vi "Configure Tag Current Pulse (Linear).vi"(0 "VISA resource name":refnum<visa-resource-name>, 1 "Source Measure Unit Channel (0: Channel A)":i32(ring) items=["Channel A", "Channel B"], 2 "Bias Level (0 A)":dbl, 3 "Voltage Limit (1 V)":dbl=1.0, 4 "Voltage Buffer (smua.nvbuffer1)":string="smua.nvbuffer1", 5 "Pulse Start Level (0.01 A)":dbl=0.01, 6 "Pulse Stop Level (0.1 A)":dbl=0.1, 7 "error in (no error)":errorcluster, 8 "Pulse Train Tag (1)":i32=1, 9 "Pulse On Time (0.02 S)":dbl=0.02, 10 "Pulse Measure Cycles (10)":i32=10, 11 "Pulse Off Time (0.04 S)":dbl=0.04, 12 "Trigger Input (0)":i32, 13 "Trigger Wait Time (10 S)":dbl=10.0, 14 "Trigger Output (0)":i32, 15 "Missing Trigger (0: Nil)":i32(ring) items=["Nil", "Abort Pulse", "Not Abort Pulse"]) -> (20 "VISA resource name out":refnum<visa-resource-name>, 27 "error out":errorcluster)   [LabVIEW 2020, in "Keithley 2600 Series.lvlib"]
doc: "Configures a linear pulsed current sweep with a voltage measurement.\n\n<b>Note:</b>\nThis VI does not cause the specified source measure unit channel to output a pulse train. It simply checks to see if all the pulse dimensions can be achieved, and if they are, assigns the indicated pulse train tag to the pulse train. You need to call <b>Initiate Pulse Test </b>VI to initiate a pulse train."
uses:
  <instrlib>/Keithley 2600 Series/Keithley 2600 Series.lvlib
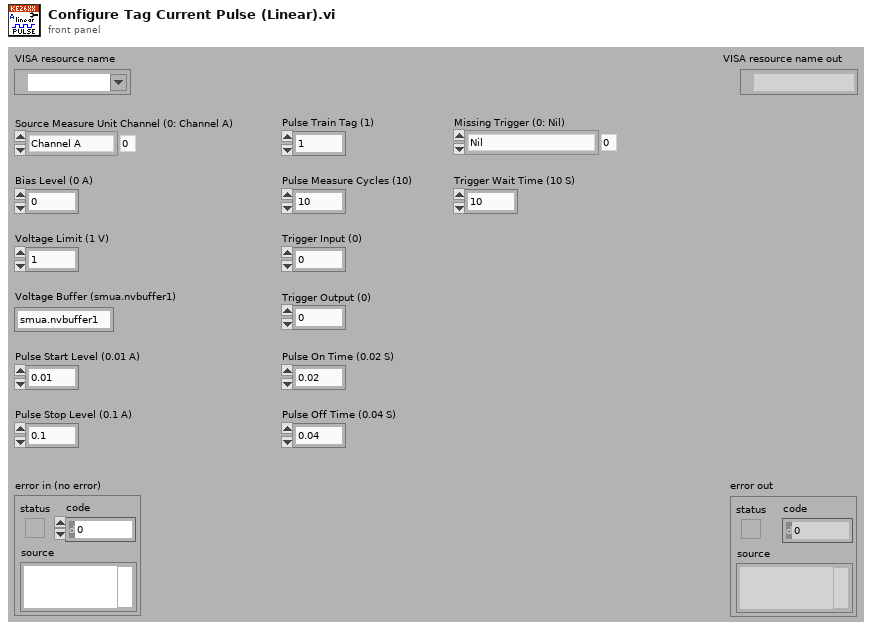
[diagram p1: front panel]
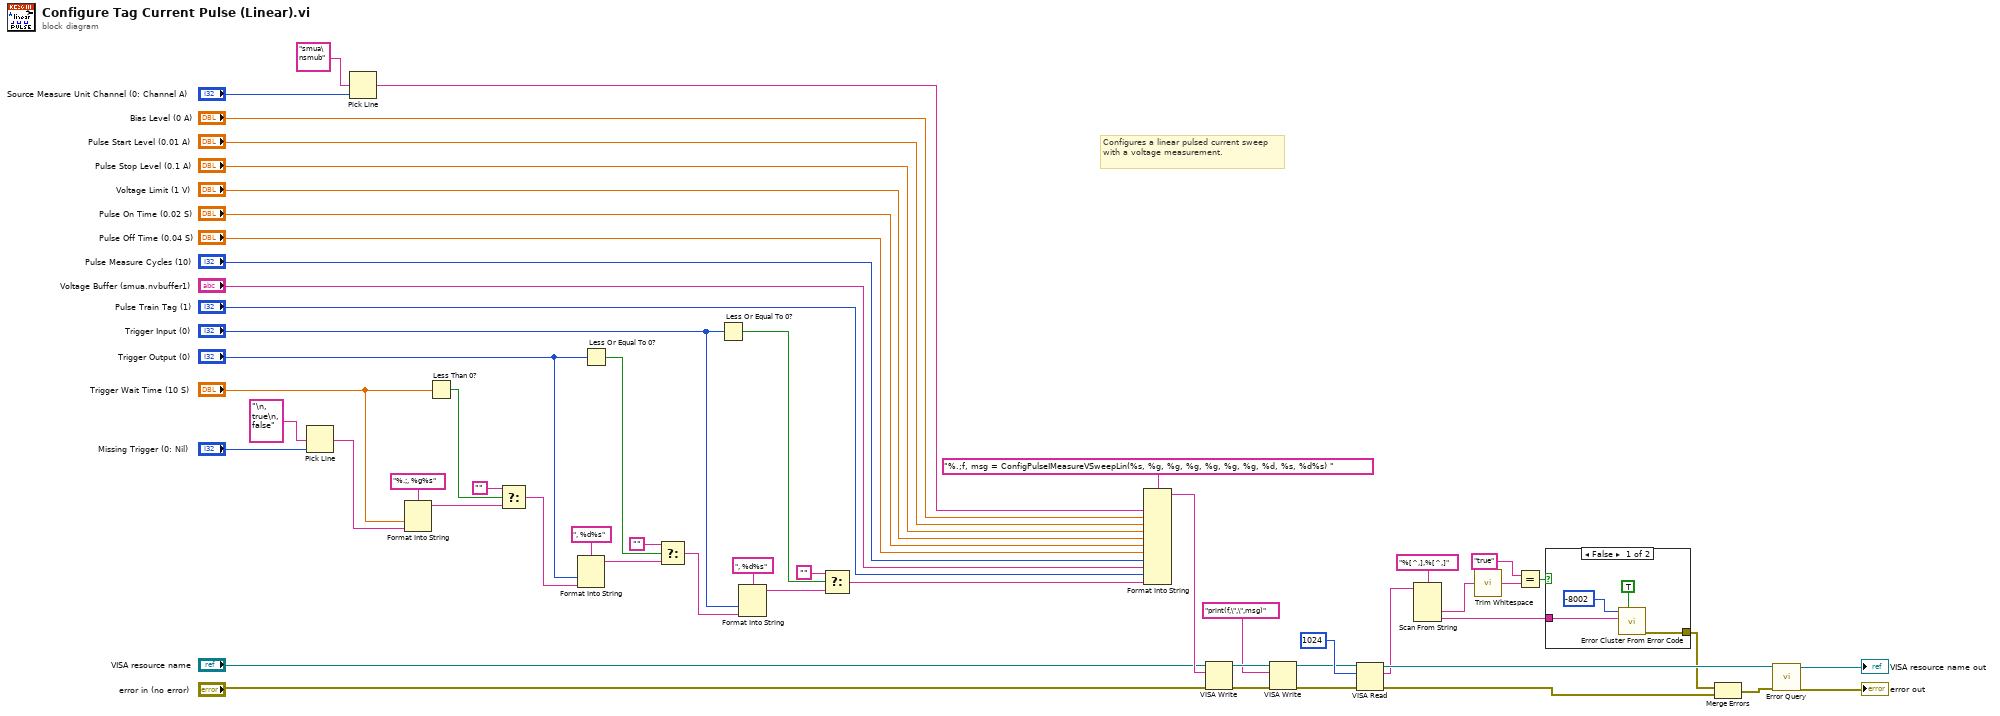
[diagram p0: block diagram]
diagram:
  # "Configures a linear pulsed current sweep with a voltage measurement."
  n1 = Pick Line(multi-line string="\n, true\n, false", line index="Missing Trigger (0: Nil)") -> (output string=w18:string)  [unwired: 1 in]
  n2 = Pick Line(multi-line string="smua\nsmub", line index="Source Measure Unit Channel (0: Channel A)") -> (output string=w15:string)  [unwired: 1 in]
  n3 = Format Into String(format string="%.;, %g%s", "Trigger Wait Time (10 S)", w18) -> (resulting string=w22:string)  [unwired: 2 in, 1 out]
  n4 = Less Than 0?(x="Trigger Wait Time (10 S)") -> (x < 0?=w28:bool)
  n5 = Select(t="", s=w28, f=w22) -> (s? t:f=w19:string)
  n6 = Format Into String(format string=", %d%s", "Trigger Output (0)", w19) -> (resulting string=w24:string)  [unwired: 2 in, 1 out]
  n7 = Less Or Equal To 0?(x="Trigger Output (0)") -> (x <= 0?=w30:bool)
  n8 = Select(t="", s=w30, f=w24) -> (s? t:f=w20:string)
  n9 = Less Or Equal To 0?(x="Trigger Input (0)") -> (x <= 0?=w32:bool)
  n10 = Format Into String(format string=", %d%s", "Trigger Input (0)", w20) -> (resulting string=w21:string)  [unwired: 2 in, 1 out]
  n11 = Select(t="", s=w32, f=w21) -> (s? t:f=w14:string)
  n12 = Format Into String(format string="%.;f, msg = ConfigPulseIMeasureVSweepLin(%s, %g, %g, %g, %g, %g, %g, %d, %s, %d%s) ", w15, "Bias Level (0 A)", "Pulse Start Level (0.01 A)", "Pulse Stop Level (0.1 A)", "Voltage Limit (1 V)", "Pulse On Time (0.02 S)", "Pulse Off Time (0.04 S)", "Pulse Measure Cycles (10)", "Voltage Buffer (smua.nvbuffer1)", "Pulse Train Tag (1)", w14) -> (resulting string=w55:string)  [unwired: 2 in, 1 out]
  n13 = VISA Write(VISA resource name="VISA resource name", write buffer=w55, error in (no error)="error in (no error)") -> (VISA resource name out=w40:refnum<visa-resource-name>, error out=w39:errorcluster)  [unwired: 1 out]
  n14 = VISA Write(VISA resource name=w40, write buffer="print(f,\",\",msg)", error in (no error)=w39) -> (VISA resource name out=w38:refnum<visa-resource-name>, error out=w37:errorcluster)  [unwired: 1 out]
  n15 = VISA Read(VISA resource name=w38, byte count=u32 1024, error in (no error)=w37) -> (VISA resource name out=w50:refnum<visa-resource-name>, read buffer=w48:string, error out=w34:errorcluster)  [unwired: 1 out]
  n16 = Scan From String(format string="%[^,],%[^,]", input string=w48) -> (output 1=w46:string, output 2=w42:string)  [unwired: 4 in, 3 out]
  n17 = call <vilib>:"Trim Whitespace.vi"("string"=w46) -> ("trimmed string"=w45:string)  [unwired: 1 in]
  n18 = Equal?(x="true", y=w45) -> (x = y?=w43:bool)
  n19 = case shown="False" w43 {
    tunnel: [w58 _] -> w35
    tunnel: w42 -> [w60 _]
    frame False {
      n20 = call <vilib>:"Error Cluster From Error Code.vi"("show call chain? (False)"=TRUE, "error message (\"\")"=w60, "error code (0)"=-8002) -> ("error out"=w58:errorcluster)  [unwired: 6 in]
    }
    frame True {
    }
  }
  n21 = Merge Errors(w35, w34) -> (w41:errorcluster)
  n22 = call <instrlib>:"Error Query.vi"("error in (no error)"=w41, "VISA resource name"=w50) -> ("error out"=→"error out":errorcluster, "VISA resource name out"=→"VISA resource name out":refnum<visa-resource-name>)  [unwired: 6 in, 2 out]
